vi "lua_replace.vi"(8 "error in (no error)":errorcluster, 10 "index":i32, 11 "lua_state_p":u64) -> (0 "error out":errorcluster, 3 "lua_state_p out":u64)   [LabVIEW 2020, in "lua.dll.lvlib"]
uses:
  lua.dll.lvlib
  lua_settop.vi
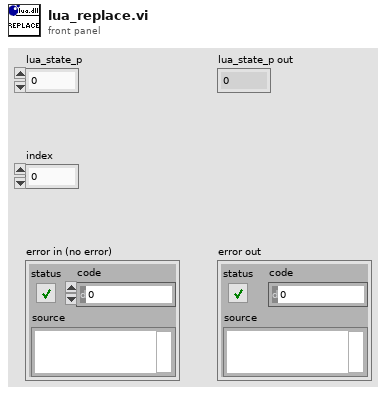
[diagram p1: front panel]
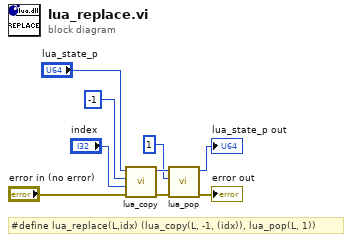
[diagram p0: block diagram]
diagram:
  # "#define lua_replace(L,idx)\t(lua_copy(L, -1, (idx)), lua_pop(L, 1))"
  n1 = call "lua_copy.vi"("error in (no error)"="error in (no error)", "toidx"="index", "fromidx"=-1, "lua_state_p"="lua_state_p") -> ("error out"=w7:errorcluster, "lua_state_p out"=w8:u64)  [unwired: 6 in]
  n2 = call "lua_pop.vi"("error in (no error)"=w7, "n"=1, "lua_state_p"=w8) -> ("error out"=→"error out":errorcluster, "lua_state_p out"=→"lua_state_p out":u64)  [unwired: 7 in]
